vi "MathCAD design.vi"(6 "MCAD file cmd":T3, 8 "error in (no error)":errorcluster, 11 "Design inputs":variant) -> (0 "error out":errorcluster)   [LabVIEW 2015, in "AguaClara Library.lvlib"]
uses:
  AguaClara Library.lvlib
  MCAD design cmds.ctl
  <vilib>/Utility/miscctls.llb/LVBoundsTypeDef.ctl
  Basic Inputs.ctl
panel:
  in  "Design Inputs":T1={"Q.Plant"=0.0033333333333333335, "C.CoagDoseMax"=0.0, "C.CoagStock"=0.0, "Ti.CoagStock"=0.0, "EN.DrillSeries"=enum."English", "EN.TubeSeries"=enum."English", "N.SedTanks"=0.0, "N.SedBaysEst"=0.0, "W.SedPlate"=0.0, "L.SedPlateSheet"=0.0, "T.SedPlate"=0.03, "T.PlantWall"=0.0254, "H.FlocOption"=0.0003, "T.FlocBaffleRigidH"=0.3, "T.ConcreteMin"=0.04, "T.SedWeir"=108000.0, "T.FlocBaffleRigidV"=0.05} {"T.FlocBaffleRigidV" min=0.001 max=0.2 step=0.001 format="%#.1f"; "T.SedWeir" min=0.005 max=0.2 step=0.001 format="%#.1f"; "T.SedPlate" min=0.3 max=8.0 step=0.01 format="%#.1f"; "T.FlocBaffleRigidH" min=0.5 max=4.0 step=0.01 format="%#.2f"; "T.ConcreteMin" min=0.0 max=0.2 step=0.001 format="%#.1f"; "L.SedPlateSheet" min=0.5 max=3.0 step=0.001 format="%#.1f"; "N.SedBaysEst" min=1.0 max=20.0 step=1.0 format="%#.0f"; "N.SedTanks" format="%#.0f"; "Ti.CoagStock" min=43200.0 max=360000.0 step=3600.0 format="%#.1f"; "H.FlocOption" min=0.05 max=0.5 step=0.001 format="%#.1f"; "C.CoagStock" min=50.0 max=500.0 step=1.0 format="%#.0f"; "C.CoagDoseMax" min=0.03 max=0.2 step=0.005 format="%#.0f"; "Q.Plant" min=0.001 max=0.2 step=0.0001 format="%#.1f"; "T.PlantWall" min=0.001 max=0.05 step=0.001 format="%#.1f"; "W.SedPlate" min=0.01 max=0.2 step=0.01 format="%#.0f"}
  in  "Caption.Size":T2={"Width"=150, "Height"=30}
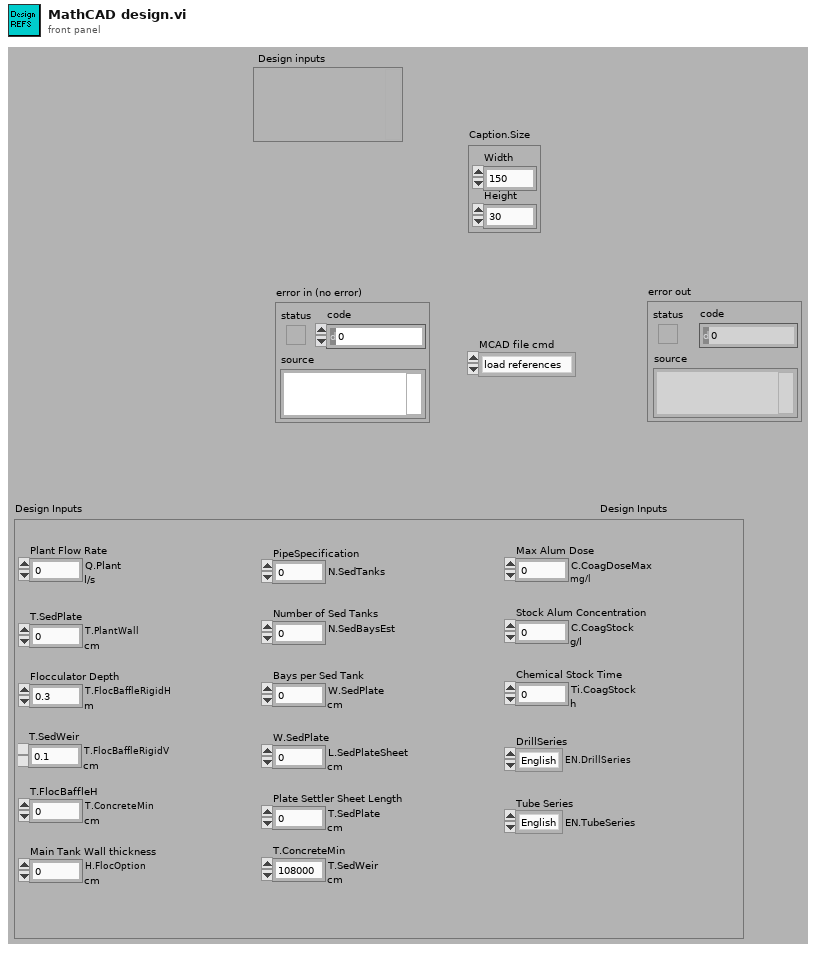
[diagram p1: front panel]
types:
  T1 = typedef "AguaClara Library.lvlib/Basic Inputs.ctl" = cluster{"Q.Plant":dbl[unit], "C.CoagDoseMax":dbl[unit], "C.CoagStock":dbl[unit], "Ti.CoagStock":dbl[unit], "EN.DrillSeries":enum16{"English", "Metric"}, "EN.TubeSeries":enum16{"English", "Metric"}, "N.SedTanks":dbl, "N.SedBaysEst":dbl, "W.SedPlate":dbl[unit], "L.SedPlateSheet":dbl[unit], "T.SedPlate":dbl[unit], "T.PlantWall":dbl[unit], "H.FlocOption":dbl[unit], "T.FlocBaffleRigidH":dbl[unit], "T.ConcreteMin":dbl[unit], "T.SedWeir":dbl[unit], "T.FlocBaffleRigidV":dbl[unit]}
  T2 = typedef "LVBoundsTypeDef.ctl" = cluster{"Width":u32, "Height":u32}
  T3 = typedef "AguaClara Library.lvlib/MCAD design cmds.ctl" = enum16{"load references", "read references"}
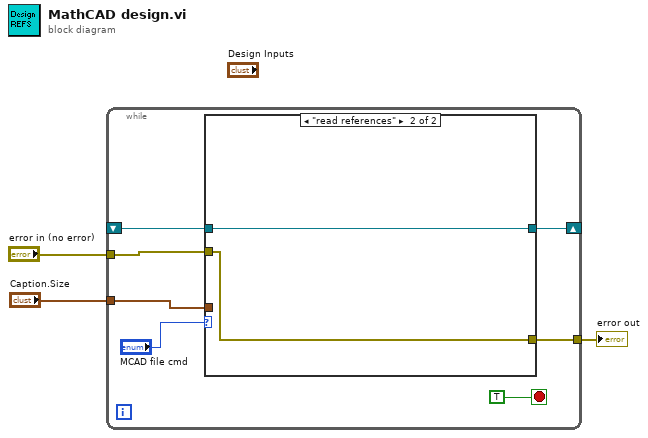
[diagram p0: block diagram]
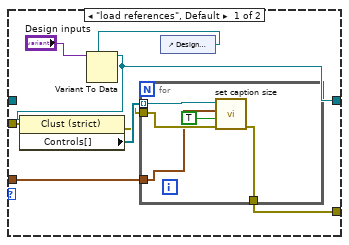
[diagram p2: hidden frame]
diagram:
  n1 = while {
    tunnel: [w8] -> w3
    tunnel: "error in (no error)" -> [w5]
    shift-right: [w7] -> _
    shift-left: _ -> [w6]
    tunnel: "Caption.Size" -> [w4]
    stop <- TRUE stop-if-true
    n2 = case shown="\"read references\"" "MCAD file cmd" {
      tunnel: [w11 w24] -> w8
      tunnel: [w12 w25] -> w7
      tunnel: w6 -> [_ w25]
      tunnel: w5 -> [w15 w24]
      tunnel: w4 -> [w17 _]
      frame "load references", Default {
        n3 = control-ref of="Design Inputs"() -> (w13:refnum<vi>)
        n4 = Variant To Data(type=w13, Variant="Design inputs") -> (data=w12:refnum<vi>)  [unwired: 1 in, 1 out]
        n5 = property class="Clust (strict)"(reference=w12, error in=w15) -> (error out=w16:errorcluster, "Controls[]"=w18:refnum<vi>[])  [unwired: 1 out]
        n6 = for {
          tunnel: w16 -> [w22]
          tunnel: w18 -> [w23] mode=indexing
          tunnel: w17 -> [w21]
          tunnel: [w19] -> w11
          n7 = call "set caption size.vi"("error in (no error)"=w22, "control visible"=TRUE, "Caption.Size"=w21, "Ctl Refnum in"=w23) -> ("error out"=w19:errorcluster)  [unwired: 6 in, 1 out]
        }
      }
      frame "read references" {
      }
    }
  }
  "error out" <- w3
